vi "AddFilter.vi"(8 "Error in (no error)":errorcluster, 10 "LogFilterInterface in":refnum<class "LogFilterInterface.lvclass">, 11 "Log in":refnum<class "Log.lvclass">) -> (0 "Error out":errorcluster, 3 "Log out":refnum<class "Log.lvclass">)   [LabVIEW 2011, in "Log.lvclass"]
uses:
  Log.lvclass
  Filter/LogFilterInterface/LogFilterInterface.lvclass
  Log.lvclass/Log.ctl
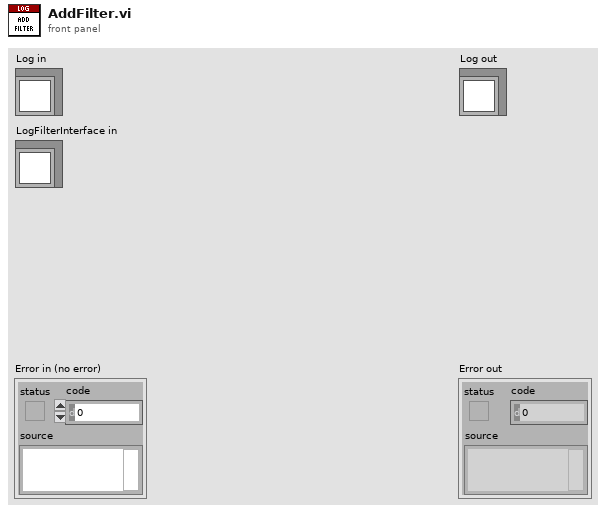
[diagram p1: front panel]
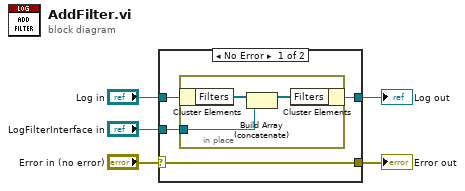
[diagram p0: block diagram]
diagram:
  n1 = case shown="No Error" "Error in (no error)" {
    selector: "Error in (no error)" -> [w9 w13]
    tunnel: [w9 w13] -> w4
    tunnel: [w6 w14] -> w2
    tunnel: "Log in" -> [w8 w14]
    tunnel: "LogFilterInterface in" -> [w7 _]
    frame No Error {
      n2 = in-place {
        in-place-border: w7 -> [w11]
        n3 = in-place-cluster #1(w8) -> ("Filters"=w12:refnum<class "LogFilterInterface.lvclass">[])
        n4 = Build Array (concatenate)(w12, w11) -> (w10:refnum<class "LogFilterInterface.lvclass">[])
        n5 = in-place-cluster #1("Filters"=w10) -> (w6:refnum<class "Log.lvclass">)
      }
    }
    frame Error {
    }
  }
  "Error out" <- w4
  "Log out" <- w2
